vi "ArrayToString.vi"(1 "Array":string[](array[string])) -> (0 "string":string)   [LabVIEW 2016]
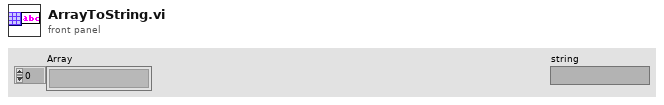
[diagram p1: front panel]
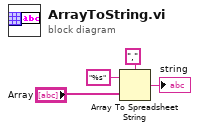
[diagram p0: block diagram]
diagram:
  n1 = Array To Spreadsheet String(delimiter (Tab)=",", array="Array", 3:"%s" ("format string")) -> (spreadsheet string=→"string":string)
